vi "New Recipe Window.vi"(8 "error in (no error)":errorcluster, 11 "Main Window in":refnum<class "Main Window.lvclass">) -> (0 "error out":errorcluster, 3 "Main Window out":refnum<class "Main Window.lvclass">)   [LabVIEW 2021, in "Recipe.lvlib" / "Main Window.lvclass"]
uses:
  Main Window.lvclass
  C:/Program Files (x86)/National Instruments/LabVIEW 2021/vi.lib/MGI/Panel Manager/Panel Actor/Panel Actor/Panel Actor.lvclass
  Recipe Window/Recipe Window.lvclass
  Main Window.lvclass/Main Window.ctl
  Recipe Window/Recipe Window.lvclass/Recipe Window.ctl
  <vilib>/MGI/Panel Manager/Panel/Panel/Subpanel/Subpanel.lvclass
  C:/Program Files (x86)/National Instruments/LabVIEW 2021/vi.lib/MGI/Panel Manager/Panel/Panel/Panel.lvclass
  <vilib>/MGI/Panel Manager/Panel/Panel/Subpanel/Subpanel.vi
  <vilib>/MGI/Panel Manager/Panel Actor/Panel Actor/Panel Actor.lvclass
  <vilib>/MGI/Panel Manager/Panel/Panel.lvlib
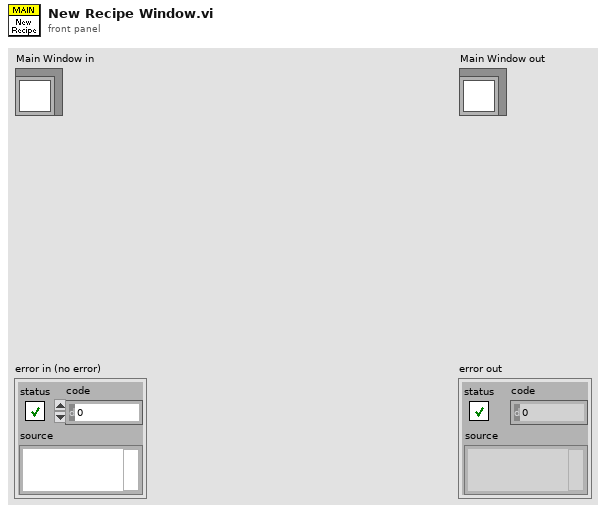
[diagram p1: front panel]
types:
  T1 = map{string, refnum<class "Message Enqueuer.lvclass">}
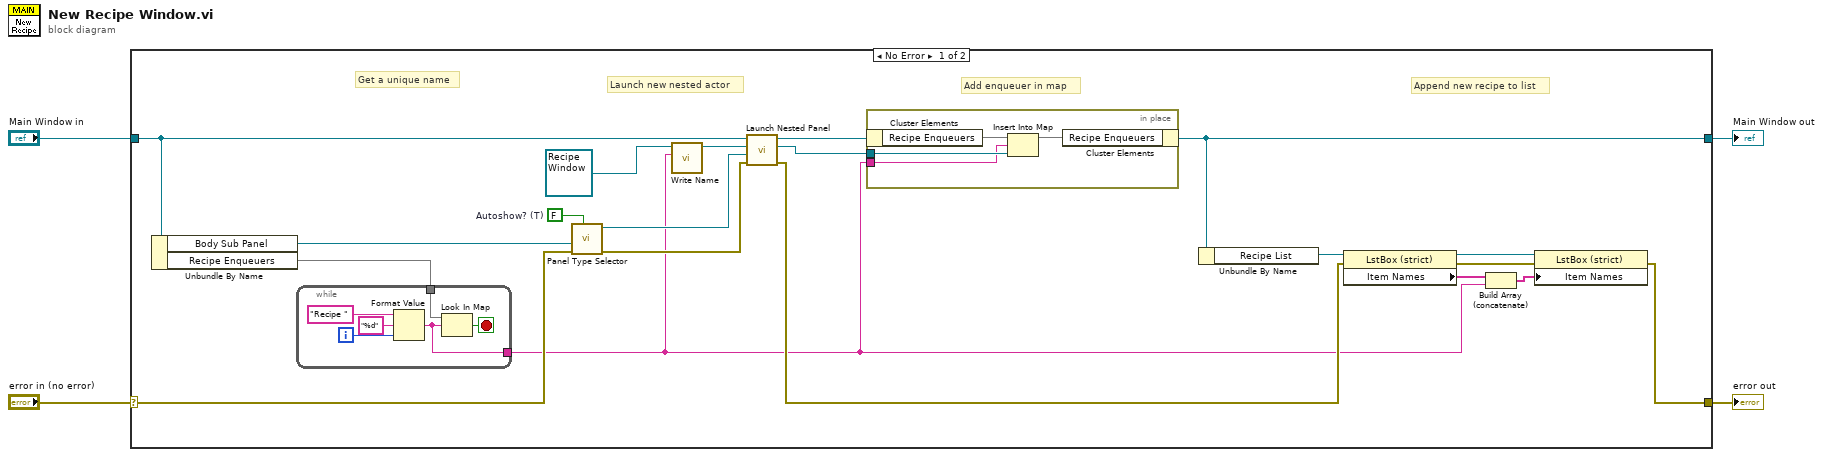
[diagram p0: block diagram]
diagram:
  n1 = case shown="No Error" "error in (no error)" {
    selector: "error in (no error)" -> [w21 w36]
    tunnel: [w14 w36] -> w3
    tunnel: [w12 w35] -> w1
    tunnel: "Main Window in" -> [w24 w35]
    frame No Error {
      w20 = FALSE  # Autoshow? (T)
      # "Append new recipe to list"
      # "Get a unique name"
      # "Add enqueuer in map"
      # "Launch new nested actor"
      n2 = Unbundle By Name(w24) -> ("Body Sub Panel"=w23:refnum<vi>, "Recipe Enqueuers"=w11:T1)
      n3 = while {
        tunnel: [w27] -> w6
        tunnel: w11 -> [w25]
        i -> [w28]
        stop <- w26 stop-if-true
        n4 = Format Value(string ("")="Recipe ", format string="%d", value (0)=w28) -> (output string=w27:string)
        n5 = Look In Map(map=w25, key=w27) -> (key not found?=w26:bool)  [unwired: 1 in, 1 out]
      }
      n6 = call-poly <vilib>:"Panel Type Selector.vi"("Autoshow? (T)"=w20, "Error In"=w21, "Sub Panel"=w23) -> ("Error Out"=w10:errorcluster, "Subpanel Out"=w22:refnum<class "Subpanel.lvclass">)  [unwired: 7 in]
      n7 = call "Write Name.vi"("Name"=w6, "Recipe Window in"=refnum<class "Recipe Window.lvclass"> refnum ("Recipe.lvlib:Recipe Window.lvclass")) -> ("Recipe Window out"=w5:refnum<class "Recipe Window.lvclass">)  [unwired: 8 in, 1 out]
      n8 = call <vilib>:"Launch Nested Panel.vi"("error in (no error)"=w10, "Panel"=w22, "Nested Panel Actor"=w5, "Panel Actor in"=w24) -> ("error out"=w7:errorcluster, "Nested Actor's Enqueuer"=w8:refnum<class "Message Enqueuer.lvclass">, "Panel Actor out"=w13:refnum<class "Main Window.lvclass">)  [unwired: 4 in, 1 out]
      n9 = in-place {
        in-place-border: w8 -> [w33]
        in-place-border: w6 -> [w31]
        n10 = in-place-cluster #1(w13) -> ("Recipe Enqueuers"=w32:T1)
        n11 = Insert Into Map(map in=w32, key=w31, value=w33) -> (map out=w34:T1)  [unwired: 2 out]
        n12 = in-place-cluster #1("Recipe Enqueuers"=w34) -> (w12:refnum<class "Main Window.lvclass">)
      }
      n13 = Unbundle By Name(w12) -> ("Recipe List"=w19:refnum<vi>)
      n14 = property class="LstBox (strict)"(reference=w19, error in=w7) -> (reference out=w18:refnum<vi>, error out=w15:errorcluster, "Item Names"=w17:string[])
      n15 = Build Array (concatenate)(w17, w6) -> (w16:string[])
      n16 = property class="LstBox (strict)"(reference=w18, error in=w15, "Item Names"=w16) -> (error out=w14:errorcluster)  [unwired: 1 out]
    }
    frame Error {
    }
  }
  "error out" <- w3
  "Main Window out" <- w1
